vi "Hardware - Setup and Arm Counter Task Jason_org.vi"(1 "error in":errorcluster) -> (0 "error out":errorcluster)   [LabVIEW 2010, in "Core SubVIs.lvlib"]
uses:
  Core SubVIs.lvlib
  Controls/TYPE - Count Time Method.ctl
  Program Files/National Instruments/LabVIEW 2010/resource/objmgr/daqmx.rc
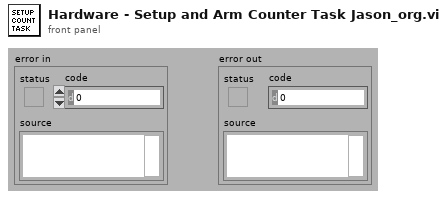
[diagram p1: front panel]
types:
  T1 = typedef "Core SubVIs.lvlib/TYPE - Count Time Method.ctl" = enum16{"Start Timer Task", "Read Timer", "Reset Timer", "Clear Timer Task"}
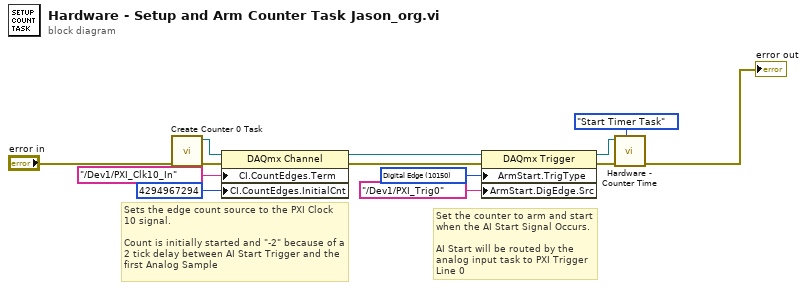
[diagram p0: block diagram]
diagram:
  w7 = 10150 items=["Digital Edge"=10150, "None"=10230] ("ArmStart.TrigType")
  # "Set the counter to arm and start when the AI Start Signal Occurs.\n\nAI Start will be routed by the analog input task to PXI Trigger Line 0"
  # "Sets the edge count source to the PXI Clock 10 signal.\n\nCount is initially started and \"-2\" because of a 2 tick delay between AI Start Trigger and the first Analog Sample"
  n1 = call "Create Counter 0 Task.vi"("error in"="error in") -> ("error out"=w3:errorcluster, "task out"=w2:refnum<k21>)  [unwired: 9 in]
  n2 = property class="DAQmx Channel"(reference=w2, error in=w3, "CI.CountEdges.Term"=tag "/Dev1/PXI_Clk10_In", "CI.CountEdges.InitialCnt"=u32 4294967294) -> (reference out=w4:refnum<k21>, error out=w5:errorcluster)
  n3 = property class="DAQmx Trigger"(reference=w4, error in=w5, "ArmStart.TrigType"=w7, "ArmStart.DigEdge.Src"=tag "/Dev1/PXI_Trig0" ("source")) -> (reference out=w10:refnum<k21>, error out=w11:errorcluster)
  n4 = call "Hardware - Counter Time.vi"("Counter Time Function (Read Timer)"=TYPE_-_Count_Time_Method."Start Timer Task", "error in (no error)"=w11, "Counter Task In"=w10) -> ("error out"=→"error out":errorcluster)  [unwired: 7 in, 1 out]
